vi "log message.vi"(8 "error in (no error)":errorcluster, 9 "log level":u16(ring) items=[" STATUS ", " DEBBUG ", "  INFO  ", "WARNING ", " ERROR  ", "CRITICAL"], 10 "Message to log":string, 11 "Log File in":refnum<class "Log File.lvclass">) -> (0 "error out":errorcluster, 3 "Log File out":refnum<class "Log File.lvclass">)   [LabVIEW 2018, in "Log File.lvclass"]
uses:
  Log File.lvclass
  Log File.lvclass/Log File.ctl
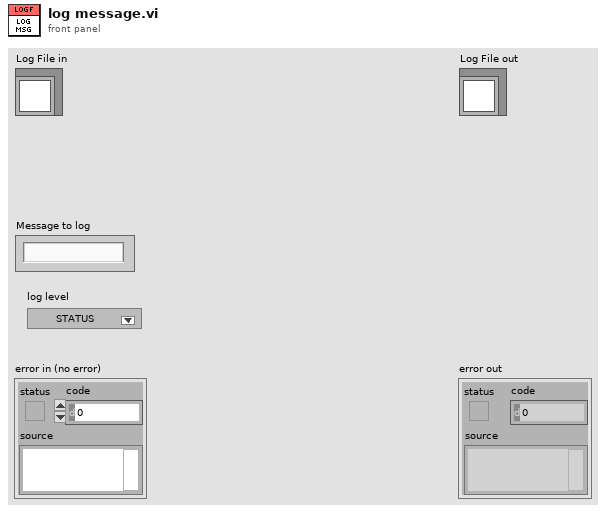
[diagram p1: front panel]
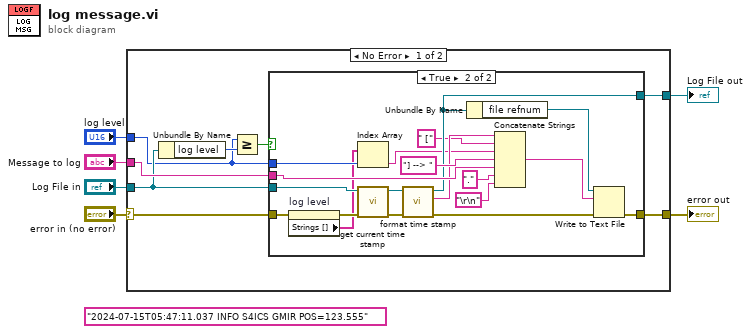
[diagram p0: block diagram]
diagram:
  (unwired) "2024-07-15T05:47:11.037 INFO S4ICS GMIR POS=123.555" ("string")
  n1 = case shown="No Error" "error in (no error)" {
    selector: "error in (no error)" -> [w12 w37]
    tunnel: [w14 w37] -> w5
    tunnel: [w9 w36] -> w3
    tunnel: "Log File in" -> [w11 w36]
    tunnel: "Message to log" -> [w13 _]
    tunnel: "log level" -> [w7 _]
    frame No Error {
      n2 = Unbundle By Name(w11) -> ("log level"=w10:u16)
      n3 = Greater Or Equal?(x=w7, y=w10) -> (x >= y?=w8:bool)
      n4 = case shown="True" w8 {
        tunnel: [w15 w35] -> w14
        tunnel: w13 -> [_ w31]
        tunnel: w12 -> [w15 w19]
        tunnel: w11 -> [w16 w26]
        tunnel: [w16 w25] -> w9
        tunnel: w7 -> [_ w23]
        frame False {
        }
        frame True {
          n5 = property on="log level" class="Ring (strict)"(error in=w19) -> (error out=w18:errorcluster, "Strings []"=w17:string[])  [unwired: 1 in, 1 out]
          n6 = Index Array(array=w17, index=w23) -> (element=w21:string)
          n7 = call "get current time stamp.vi"("error in (no error)"=w18, "Log File in"=w26) -> ("error out"=w29:errorcluster, "Log File out"=w28:refnum<class "Log File.lvclass">)  [unwired: 8 in]
          n8 = call "format time stamp.vi"("error in (no error)"=w29, "Log File in"=w28) -> ("error out"=w24:errorcluster, "current time stamp"=w27:string, "Log File out"=w25:refnum<class "Log File.lvclass">)  [unwired: 7 in]
          n9 = Unbundle By Name(w25) -> ("file refnum"=w30:refnum<file>)
          n10 = Concatenate Strings(w27, " [" ("string"), w21, "] --> " ("string"), w31, "." ("string"), "\r\n") -> (w33:string)
          n11 = Write to Text File(file (use dialog)=w30, text=w33, error in=w24) -> (error out=w35:errorcluster)  [unwired: 1 in, 2 out]
        }
      }
    }
    frame Error {
    }
  }
  "error out" <- w5
  "Log File out" <- w3
